vi "XNET.Settings.vi"(6 "Action":enum8{"Get", "Set"}(ring), 8 "error in (no error)":errorcluster, 10 "J1939 XNET Settings":T1 {"Termination" items=["Off", "On"]}, 11 "Parent Ref in":T2 format="%.0x") -> (0 "error out":errorcluster, 2 "J1939 XNET Settings":T1={"Database"="", "Cluster"="", "Port"="", "Baud rate [Bd]"=0, "Termination"=0, "Incoming Rate"=100, "Outcoming Rate"=100, "Write Decimation"=1} {"Termination" items=["Off", "On"]}, 3 "Item Ref out":T2 format="%.0x")   [LabVIEW 2015, in "J1939 Addon System Explorer.lvlib"]
uses:
  J1939 Addon System Explorer.lvlib
  Shared/Types/XNET Settings.ctl
  <vilib>/NI Veristand/Custom Device API/Custom Device Item Ref.ctl
  Shared/SubVIs/Constants.vi
  <vilib>/NI Veristand/Custom Device API/Set Item Property (String).vi
  <vilib>/NI Veristand/Custom Device API/Set Item Property (U32).vi
  <vilib>/NI Veristand/Custom Device API/Get Item Property (String).vi
  <vilib>/NI Veristand/Custom Device API/Get Item Property (U32).vi
  <vilib>/NI VeriStand/Custom Device API/Custom Device API.lvlib
  Shared/J1939 Addon Shared.lvlib
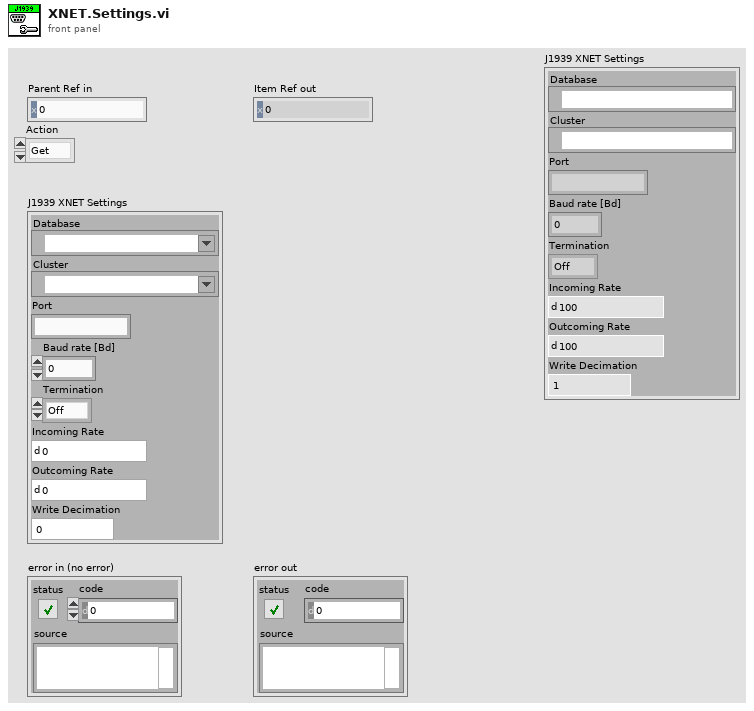
[diagram p1: front panel]
types:
  T1 = typedef "J1939 Addon Shared.lvlib/XNET Settings.ctl" = cluster{"Database":refnum<k21>, "Cluster":refnum<k21>, "Port":string, "Baud rate [Bd]":u32, "Termination":u32, "Incoming Rate":u32, "Outcoming Rate":u32, "Write Decimation":u32}
  T2 = typedef "Custom Device API.lvlib/Custom Device Item Ref.ctl" = u64
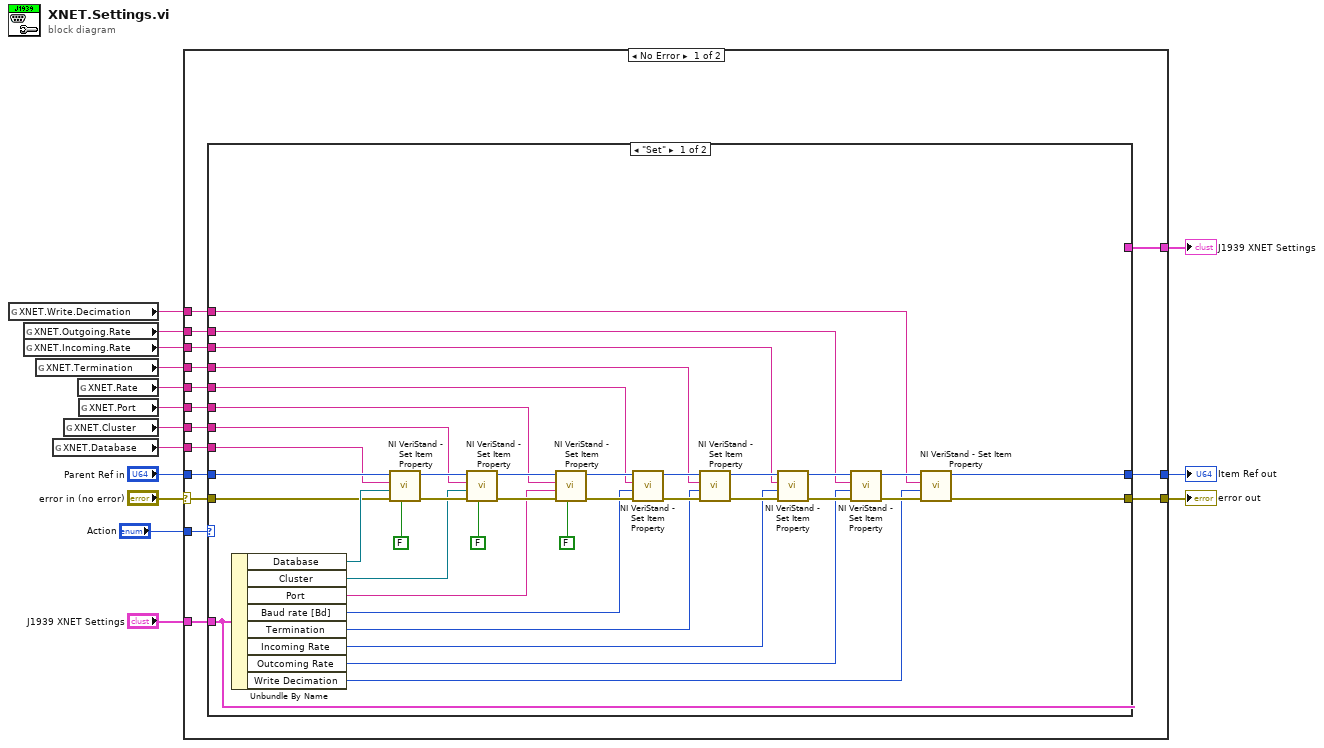
[diagram p0: block diagram]
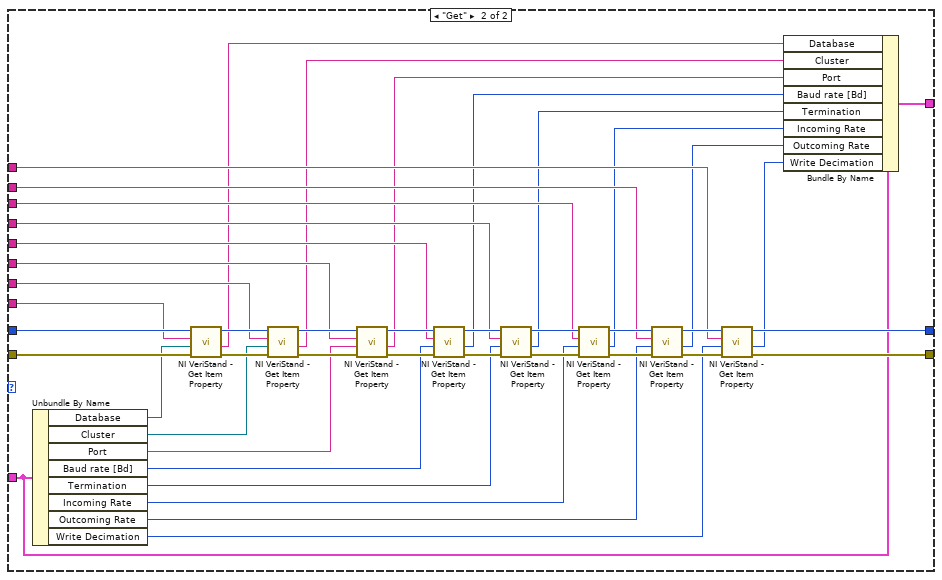
[diagram p2: hidden frame]
diagram:
  n1 = global read "Constants.vi" "XNET.Write.Decimation"() -> (w8:string)
  n2 = global read "Constants.vi" "XNET.Outgoing.Rate"() -> (w7:string)
  n3 = global read "Constants.vi" "XNET.Incoming.Rate"() -> (w6:string)
  n4 = global read "Constants.vi" "XNET.Termination"() -> (w5:string)
  n5 = global read "Constants.vi" "XNET.Database"() -> (w14:string)
  n6 = global read "Constants.vi" "XNET.Cluster"() -> (w10:string)
  n7 = global read "Constants.vi" "XNET.Rate"() -> (w4:string)
  n8 = global read "Constants.vi" "XNET.Port"() -> (w9:string)
  n9 = case shown="No Error" "error in (no error)" {
    selector: "error in (no error)" -> [w18 w115]
    tunnel: "Parent Ref in" -> [w30 w114]
    tunnel: w14 -> [w29 _]
    tunnel: "J1939 XNET Settings" -> [w28 w113]
    tunnel: [w27 w115] -> w12
    tunnel: [w26 w114] -> w11
    tunnel: w10 -> [w25 _]
    tunnel: w9 -> [w24 _]
    tunnel: w8 -> [w23 _]
    tunnel: w7 -> [w22 _]
    tunnel: w6 -> [w21 _]
    tunnel: w5 -> [w20 _]
    tunnel: w4 -> [w19 _]
    tunnel: "Action" -> [w17 _]
    tunnel: [w16 w113] -> w1
    frame No Error {
      n10 = case shown="\"Set\"" w17 {
        tunnel: w30 -> [w68 w112]
        tunnel: w29 -> [w67 w111]
        tunnel: w28 -> [w31 w78]
        tunnel: [w50 w97] -> w27
        tunnel: [w48 w95] -> w26
        tunnel: w25 -> [w39 w94]
        tunnel: w24 -> [w38 w93]
        tunnel: w23 -> [w37 w92]
        tunnel: w22 -> [w36 w91]
        tunnel: w21 -> [w35 w90]
        tunnel: w20 -> [w34 w89]
        tunnel: w19 -> [w33 w88]
        tunnel: w18 -> [w32 w87]
        tunnel: [w31 w69] -> w16
        frame "Set" {
          n11 = Unbundle By Name(w31) -> ("Database"=w47:refnum<k21>, "Cluster"=w46:refnum<k21>, "Port"=w45:string, "Baud rate [Bd]"=w44:u32, "Termination"=w43:u32, "Incoming Rate"=w42:u32, "Outcoming Rate"=w41:u32, "Write Decimation"=w40:u32)
          n12 = call-poly <vilib>:"NI VeriStand - Set Item Property.vi"("Binary String (T)"=FALSE, "error in (no error)"=w32, "Value"=w47, "Property Name"=w67, "Item Ref in"=w68) -> ("error out"=w61:errorcluster, "Item Ref out"=w60:T2)  [unwired: 4 in, 1 out]
          n13 = call-poly <vilib>:"NI VeriStand - Set Item Property.vi"("Binary String (T)"=FALSE, "error in (no error)"=w61, "Value"=w46, "Property Name"=w39, "Item Ref in"=w60) -> ("error out"=w62:errorcluster, "Item Ref out"=w63:T2)  [unwired: 4 in, 1 out]
          n14 = call-poly <vilib>:"NI VeriStand - Set Item Property.vi"("Binary String (T)"=FALSE, "error in (no error)"=w62, "Value"=w45, "Property Name"=w38, "Item Ref in"=w63) -> ("error out"=w51:errorcluster, "Item Ref out"=w49:T2)  [unwired: 4 in, 1 out]
          n15 = call-poly <vilib>:"NI VeriStand - Set Item Property.vi"("error in (no error)"=w51, "Value"=w44, "Property Name"=w33, "Item Ref in"=w49) -> ("error out"=w55:errorcluster, "Item Ref out"=w58:T2)  [unwired: 5 in, 1 out]
          n16 = call-poly <vilib>:"NI VeriStand - Set Item Property.vi"("error in (no error)"=w55, "Value"=w43, "Property Name"=w34, "Item Ref in"=w58) -> ("error out"=w54:errorcluster, "Item Ref out"=w57:T2)  [unwired: 5 in, 1 out]
          n17 = call-poly <vilib>:"NI VeriStand - Set Item Property.vi"("error in (no error)"=w54, "Value"=w42, "Property Name"=w35, "Item Ref in"=w57) -> ("error out"=w53:errorcluster, "Item Ref out"=w56:T2)  [unwired: 5 in, 1 out]
          n18 = call-poly <vilib>:"NI VeriStand - Set Item Property.vi"("error in (no error)"=w53, "Value"=w41, "Property Name"=w36, "Item Ref in"=w56) -> ("error out"=w52:errorcluster, "Item Ref out"=w59:T2)  [unwired: 5 in, 1 out]
          n19 = call-poly <vilib>:"NI VeriStand - Set Item Property.vi"("error in (no error)"=w52, "Value"=w40, "Property Name"=w37, "Item Ref in"=w59) -> ("error out"=w50:errorcluster, "Item Ref out"=w48:T2)  [unwired: 5 in, 1 out]
        }
        frame "Get" {
          n20 = Unbundle By Name(w78) -> ("Database"=w86:refnum<k21>, "Cluster"=w85:refnum<k21>, "Port"=w84:string, "Baud rate [Bd]"=w83:u32, "Termination"=w82:u32, "Incoming Rate"=w81:u32, "Outcoming Rate"=w80:u32, "Write Decimation"=w79:u32)
          n21 = call-poly <vilib>:"NI VeriStand - Get Item Property.vi"("error in (no error)"=w87, "Default Value"=w86, "Property Name"=w111, "Item Ref in"=w112) -> ("error out"=w108:errorcluster, "Value"=w77:string, "Item Ref out"=w107:T2)  [unwired: 4 in, 1 out]
          n22 = call-poly <vilib>:"NI VeriStand - Get Item Property.vi"("error in (no error)"=w108, "Default Value"=w85, "Property Name"=w94, "Item Ref in"=w107) -> ("error out"=w109:errorcluster, "Value"=w76:string, "Item Ref out"=w110:T2)  [unwired: 4 in, 1 out]
          n23 = call-poly <vilib>:"NI VeriStand - Get Item Property.vi"("error in (no error)"=w109, "Default Value"=w84, "Property Name"=w93, "Item Ref in"=w110) -> ("error out"=w98:errorcluster, "Value"=w75:string, "Item Ref out"=w96:T2)  [unwired: 4 in, 1 out]
          n24 = call-poly <vilib>:"NI VeriStand - Get Item Property.vi"("error in (no error)"=w98, "Default Value"=w83, "Property Name"=w88, "Item Ref in"=w96) -> ("error out"=w102:errorcluster, "Value"=w74:u32, "Item Ref out"=w105:T2)  [unwired: 4 in, 1 out]
          n25 = call-poly <vilib>:"NI VeriStand - Get Item Property.vi"("error in (no error)"=w102, "Default Value"=w82, "Property Name"=w89, "Item Ref in"=w105) -> ("error out"=w101:errorcluster, "Value"=w73:u32, "Item Ref out"=w104:T2)  [unwired: 4 in, 1 out]
          n26 = call-poly <vilib>:"NI VeriStand - Get Item Property.vi"("error in (no error)"=w101, "Default Value"=w81, "Property Name"=w90, "Item Ref in"=w104) -> ("error out"=w100:errorcluster, "Value"=w72:u32, "Item Ref out"=w103:T2)  [unwired: 4 in, 1 out]
          n27 = call-poly <vilib>:"NI VeriStand - Get Item Property.vi"("error in (no error)"=w100, "Default Value"=w80, "Property Name"=w91, "Item Ref in"=w103) -> ("error out"=w99:errorcluster, "Value"=w71:u32, "Item Ref out"=w106:T2)  [unwired: 4 in, 1 out]
          n28 = call-poly <vilib>:"NI VeriStand - Get Item Property.vi"("error in (no error)"=w99, "Default Value"=w79, "Property Name"=w92, "Item Ref in"=w106) -> ("error out"=w97:errorcluster, "Value"=w70:u32, "Item Ref out"=w95:T2)  [unwired: 4 in, 1 out]
          n29 = Bundle By Name(cluster=w78, "Database"=w77, "Cluster"=w76, "Port"=w75, "Baud rate [Bd]"=w74, "Termination"=w73, "Incoming Rate"=w72, "Outcoming Rate"=w71, "Write Decimation"=w70) -> (w69:T1)
        }
      }
    }
    frame Error {
    }
  }
  "Item Ref out" <- w11
  "error out" <- w12
  "J1939 XNET Settings" <- w1
